vi "CreatePrivateEvents.vi"(8 "error in (no error)":errorcluster, 11 "SMO.jsonRPC":refnum<class "SMO.jsonRPC.lvclass">) -> (0 "error out":errorcluster, 3 "SMO.jsonRPC out":refnum<class "SMO.jsonRPC.lvclass">)   [LabVIEW 2013, in "SMO.jsonRPC.lvclass"]
doc: "---------------------------------------------------------------\nJKI State Machine Objects™\nhttp://jki.net/state-machine-objects/\nCopyright (C) 2005-2015, JKI <info@jki.net>\nALL RIGHTS RESERVEDJKI State Machine Objects (SMO) 1.0.0.5\nJKI - JKI\nCopyright (c) 2016, JKI"
uses:
  SMO.jsonRPC.lvclass
  <vilib>/JKI/JKI SMO/SMO/SMO.lvclass
  SMO.jsonRPC.lvclass/SMO.jsonRPC.ctl
  Typedefs/Request--Cluster.ctl
panel:
  # "For instructions on how to use the JKI State Machine Objects, examples and video tutorials, visit:\nhttp://jki.net/state-machine-objects/\n\nJKI State Machine Objects™\nhttp://jki.net/state-machine-objects/\nCopyright (C) 2005-2015, JKI <info@jki.net>\nALL RIGHTS RESERVED"
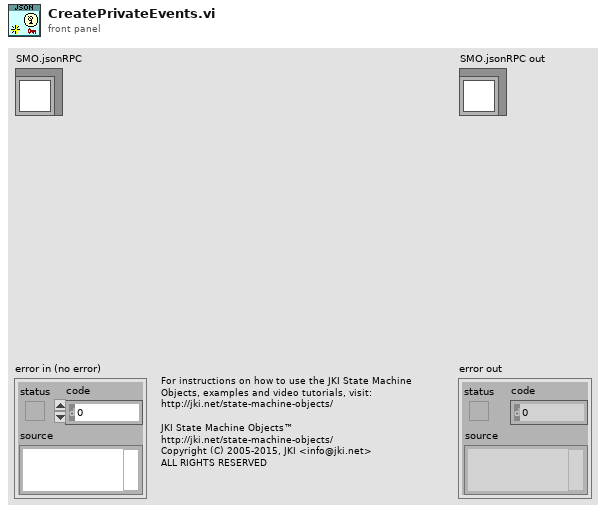
[diagram p1: front panel]
types:
  T1 = typedef "SMO.jsonRPC.lvclass/PrivateData--Ref.ctl" = refnum<data-value>
  T2 = typedef "SMO.jsonRPC.lvclass/Request--Cluster.ctl" = cluster{"Message":string, "reply queue":refnum<queue>, "Async?":bool}
  T3 = typedef "SMO.jsonRPC.lvclass/PrivateData--Cluster.ctl" = cluster{"Public Events":T4, "Private Events":T5, "Data":string}
  T4 = typedef "SMO.jsonRPC.lvclass/PublicEvents--Cluster.ctl" = cluster{"Reply":refnum<user-event>}
  T5 = typedef "SMO.jsonRPC.lvclass/PrivateEvents--Cluster.ctl" = cluster{"Incoming Request":refnum<user-event>}
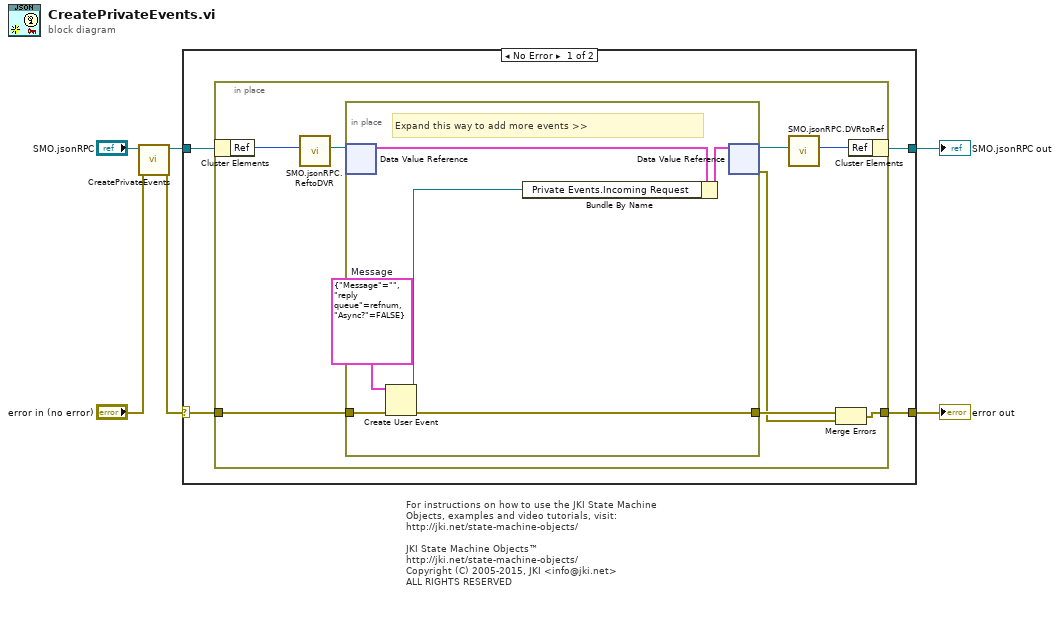
[diagram p0: block diagram]
diagram:
  # "For instructions on how to use the JKI State Machine Objects, examples and video tutorials, visit:\nhttp://jki.net/state-machine-objects/\n\nJKI State Machine Objects™\nhttp://jki.net/state-machine-objects/\nCopyright (C) 2005-2015, JKI <info@jki.net>\nALL RIGHTS RESERVED"
  n1 = call-parent "CreatePrivateEvents.vi"("error in (no error)"="error in (no error)", "SMO"="SMO.jsonRPC") -> ("error out"=w1:errorcluster, "SMO out"=w3:refnum<class "SMO.jsonRPC.lvclass">)  [unwired: 8 in]
  n2 = case shown="No Error" w1 {
    selector: w1 -> [w8 w26]
    tunnel: [w7 w26] -> w5
    tunnel: [w9 w25] -> w6
    tunnel: w3 -> [w10 w25]
    frame No Error {
      n3 = in-place {
        in-place-border: w8 -> [w18]
        in-place-border: [w15] -> w7
        n4 = in-place-cluster #1(w10) -> ("Ref"=w14:u32)
        n5 = call "SMO.jsonRPC.ReftoDVR.vi"("Ref"=w14) -> ("Ref"=w13:T1)  [unwired: 10 in]
        n6 = in-place {
          in-place-border: w18 -> [w22]
          in-place-border: [w23] -> w17
          w20 = T2 {"Message"="", "reply queue"=refnum, "Async?"=FALSE}  # Message
          # "Expand this way to add more events >>"
          n7 = in-place-dvr #2(w13) -> (w21:T3)  [unwired: 1 out]
          n8 = Create User Event(user event datatype=w20, error in=w22) -> (user event=w19:refnum<user-event>, error out=w23:errorcluster)
          n9 = Bundle By Name(cluster=w21, "Private Events.Incoming Request"=w19) -> (w24:T3)
          n10 = in-place-dvr #2(w24) -> (w12:T1, w16:errorcluster)
        }
        n11 = call "SMO.jsonRPC.DVRtoRef.vi"("Ref"=w12) -> ("Ref"=w11:u32)  [unwired: 10 in]
        n12 = Merge Errors(w17, w16) -> (w15:errorcluster)
        n13 = in-place-cluster #1("Ref"=w11) -> (w9:refnum<class "SMO.jsonRPC.lvclass">)
      }
    }
    frame Error {
    }
  }
  "error out" <- w5
  "SMO.jsonRPC out" <- w6
